vi "Main.vi"() -> ()   [LabVIEW 2014]
panel:
  out "Ones":bool[](array[boolean])
  out "Tens":bool[](array[boolean]) caption="Binary Representation"
  in  "Input":u8
  in  "Stop Button":bool
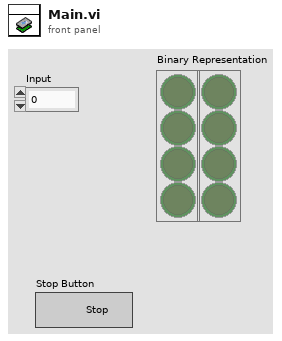
[diagram p1: front panel]
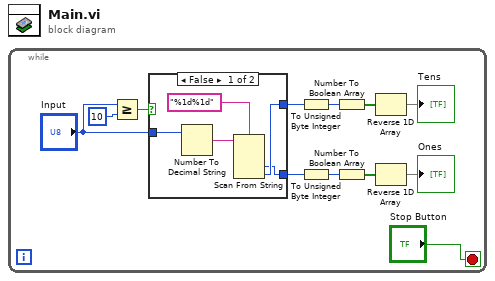
[diagram p0: block diagram]
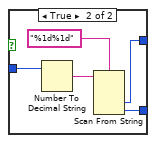
[diagram p2: hidden frame]
diagram:
  n1 = while {
    stop <- "Stop Button" stop-if-true
    n2 = Greater Or Equal?(x="Input", y=u8 10) -> (x >= y?=w11:bool)
    n3 = case shown="False" w11 {
      tunnel: "Input" -> [w16 w22]
      tunnel: [w14 w19] -> w6
      tunnel: [w13 w18] -> w3
      frame False {
        n4 = Number To Decimal String(number=w16) -> (decimal integer string=w17:string)  [unwired: 1 in]
        n5 = Scan From String(format string="%1d%1d", input string=w17) -> (output 1=w13:i32, output 2=w14:i32)  [unwired: 4 in, 3 out]
      }
      frame True {
        n6 = Number To Decimal String(number=w22) -> (decimal integer string=w21:string)  [unwired: 1 in]
        n7 = Scan From String(format string="%1d%1d", input string=w21) -> (output 1=w19:i32, output 2=w18:i32)  [unwired: 4 in, 3 out]
      }
    }
    n8 = To Unsigned Byte Integer(number=w6) -> (unsigned 8bit integer=w5:u8)
    n9 = To Unsigned Byte Integer(number=w3) -> (unsigned 8bit integer=w4:u8)
    n10 = Number To Boolean Array(number=w5) -> (Boolean array=w8:bool[])
    n11 = Number To Boolean Array(number=w4) -> (Boolean array=w7:bool[])
    n12 = Reverse 1D Array(array=w8) -> (reversed array=→"Tens":bool[])
    n13 = Reverse 1D Array(array=w7) -> (reversed array=→"Ones":bool[])
  }
